vi "HW_6p1_Task1_pipoat.vi"() -> ()   [LabVIEW 2016]
uses:
  <vilib>/express/express arith-compare/Formula/XNode/ExpressFormulaBlockNode.xnode
panel:
  out "Final (B)":dbl
  out "Final (A)":dbl
  in  "Target Concentration":dbl
  out "Concentration of C (mol/L)":dbl
  in  "Initial Value A (mol/L)":dbl
  in  "Initial Value B (mol/L)":dbl
  out "Minutes":i32
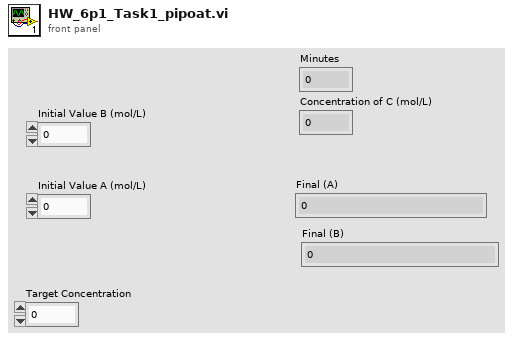
[diagram p1: front panel]
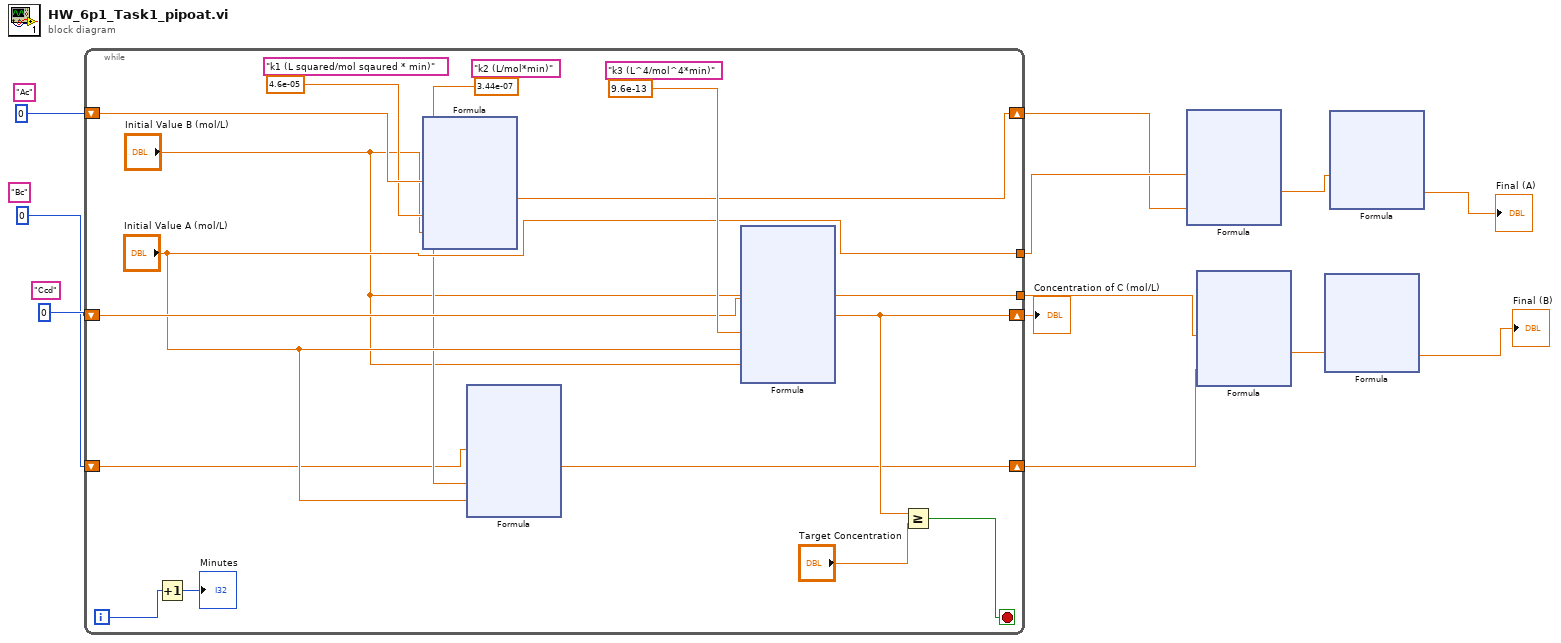
[diagram p0: block diagram]
diagram:
  (unwired) "Bc"
  (unwired) "Ccd"
  (unwired) "Ac"
  n1 = while {
    shift-right: [w16] -> w8
    shift-left: 0 -> [w25]
    shift-right: [w21] -> w10
    shift-left: 0 -> [w19]
    tunnel: ["Initial Value A (mol/L)"] -> w11
    tunnel: ["Initial Value B (mol/L)"] -> w3
    shift-right: [w14] -> w2
    shift-left: 0 -> [w13]
    i -> [w27]
    stop <- w22 stop-if-true
    (unwired) "k3 (L^4/mol^4*min)"
    (unwired) "k2 (L/mol*min)"
    (unwired) "k1 (L squared/mol sqaured * min)"
    n2 = Increment(x=w27) -> (x+1=→"Minutes":i32)
    n3 = xnode "Formula"("Ac"=w25, "k1"=4.6e-05, "Cbi"="Initial Value B (mol/L)") -> ("Result"=w16:dbl)  [unwired: 1 in, 1 out]
    n4 = xnode "Formula"("Bc"=w13, "k2"=3.44e-07, "Cai"="Initial Value A (mol/L)") -> ("Result"=w14:dbl)  [unwired: 1 in, 1 out]
    n5 = xnode "Formula"("Ccd"=w19, "k3"=9.6e-13, "Cai"="Initial Value A (mol/L)", "Cbi"="Initial Value B (mol/L)") -> ("Result"=w21:dbl)  [unwired: 1 in, 1 out]
    n6 = Greater Or Equal?(x=w21, y="Target Concentration") -> (x >= y?=w22:bool)
  }
  "Concentration of C (mol/L)" <- w10
  n7 = xnode "Formula"("Cai"=w11, "Ac"=w8) -> ("Result"=w7:dbl)  [unwired: 1 in, 1 out]
  n8 = xnode "Formula"("Cbi"=w3, "Bc"=w2) -> ("Result"=w4:dbl)  [unwired: 1 in, 1 out]
  n9 = xnode "Formula"("Cbi"=w4) -> ("Result"=→"Final (B)":dbl)  [unwired: 1 in, 1 out]
  n10 = xnode "Formula"("Cai"=w7) -> ("Result"=→"Final (A)":dbl)  [unwired: 1 in, 1 out]
